vi "Agilent DSO1000 Series Acquire Waveform.vi"() -> ()   [LabVIEW 2010]
doc: "This example shows how to use autosetup and acquire a waveform on a single channel."
uses:
  <instrlib>/Agilent DSO1000 Series/Public/Data/Read Waveform (Single).vi
  <instrlib>/Agilent DSO1000 Series/Agilent DSO1000 Series.lvlib
panel:
  in  "Channel (1: Channel 1)":u16(ring)=1 items=["Channel 1"=1, "Channel 2"=2, "Channel 3"=3, "Channel 4"=4]
  in  "Maximum Time (10000 ms)":u32=10000
  in  "Probe Attenuation (10.0)":dbl=10.0
  out "Waveform Data":waveform(dbl)(graph)
  in  "VISA resource name":refnum<visa-resource-name>
  # "(c) 2009 National Instruments.  ALL RIGHTS RESERVED."
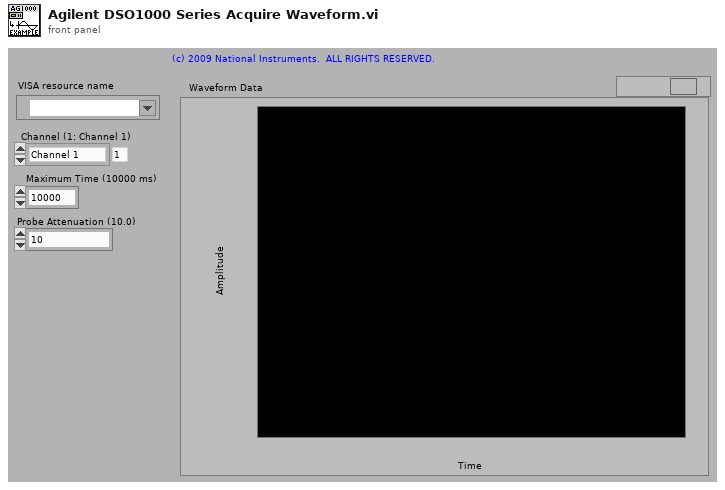
[diagram p1: front panel]
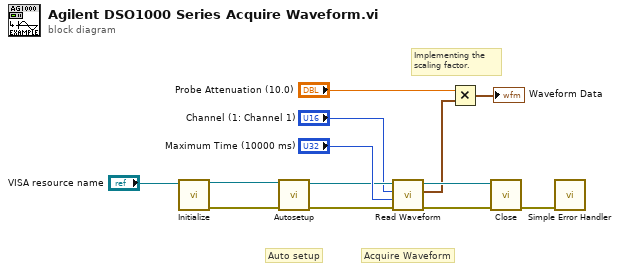
[diagram p0: block diagram]
diagram:
  # "Implementing the \nscaling factor."
  # "Acquire Waveform"
  # "Auto setup"
  n1 = call <instrlib>:"Initialize.vi"("VISA resource name"="VISA resource name") -> ("error out"=w11:errorcluster, "VISA resource name out"=w10:refnum<visa-resource-name>)  [unwired: 9 in]
  n2 = call <instrlib>:"Autosetup.vi"("error in (no error)"=w11, "VISA resource name"=w10) -> ("error out"=w2:errorcluster, "VISA resource name out"=w3:refnum<visa-resource-name>)  [unwired: 8 in]
  n3 = call-poly <instrlib>:"Read Waveform.vi"("error in (no error)"=w2, "Maximum Time (10000 ms)"="Maximum Time (10000 ms)", "Channel (1: Channel 1)"="Channel (1: Channel 1)", "VISA resource name"=w3) -> ("error out"=w5:errorcluster, "Waveform Data"=w6:waveform(dbl), "VISA resource name out"=w7:refnum<visa-resource-name>)  [unwired: 5 in]
  n4 = Multiply(x="Probe Attenuation (10.0)", y=w6) -> (x*y=→"Waveform Data":waveform(dbl))
  n5 = call <instrlib>:"Close.vi"("error in (no error)"=w5, "VISA resource name"=w7) -> ("error out"=w13:errorcluster)  [unwired: 9 in]
  n6 = call <vilib>:"Simple Error Handler.vi"("error in (no error)"=w13) -> ()  [unwired: 4 in, 5 out]
